vi "Set Tile.vi"(8 "error in (no error)":errorcluster, 10 "Tile":bool[][](array[boolean]), 11 "Tile in":refnum<class "Tile.lvclass">) -> (0 "error out":errorcluster, 3 "Tile out":refnum<class "Tile.lvclass">)   [LabVIEW 2020, in "Tile.lvclass"]
uses:
  Tile.lvclass
  Tile.lvclass/Tile.ctl
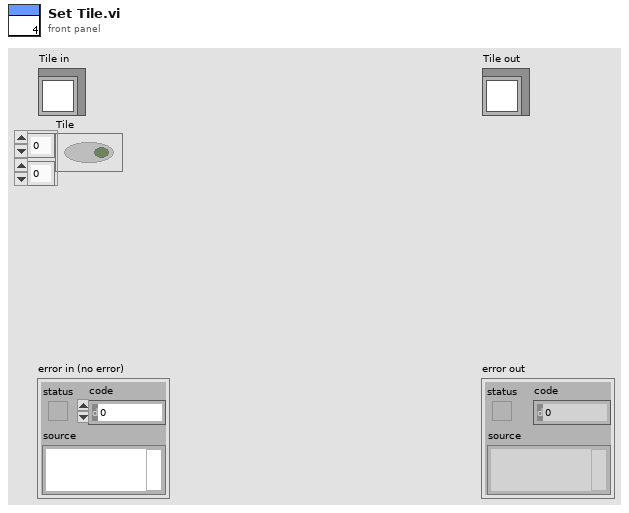
[diagram p1: front panel]
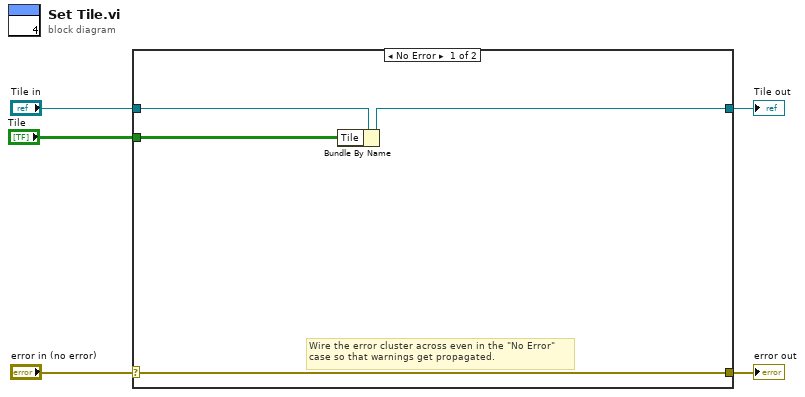
[diagram p0: block diagram]
diagram:
  n1 = case shown="No Error" "error in (no error)" {
    selector: "error in (no error)" -> [w9 w11]
    tunnel: [w9 w11] -> w4
    tunnel: [w8 w10] -> w2
    tunnel: "Tile in" -> [w7 w10]
    tunnel: "Tile" -> [w6 _]
    frame No Error {
      # "Wire the error cluster across even in the \"No Error\"\ncase so that warnings get propagated."
      n2 = Bundle By Name(cluster=w7, "Tile"=w6) -> (w8:refnum<class "Tile.lvclass">)
    }
    frame Error {
    }
  }
  "error out" <- w4
  "Tile out" <- w2
